vi "9234_Initialize.vi"(8 "error in (no error)":errorcluster, 9 "Slot Settings":T1, 11 "9234 in":refnum<class "9234.lvclass">) -> (0 "error out":errorcluster, 3 "9234 out":refnum<class "9234.lvclass">)   [LabVIEW 2017, in "Modules.lvlib" / "9234.lvclass"]
uses:
  9234.lvclass
  RSI Module/Slot Settings.ctl
  C:/Users/dbuck/Documents/GitHub/Scan-Engine-Custom-Device-Classes/Source/RSI Module/RSI Module.lvclass
  RSI Module/Channels.ctl
  RSI Module/Channel Type.ctl
  RSI Module/Module Models.ctl
  Data rate.ctl
  9234.lvclass/9234.ctl
  RSI Module/RSI Module.lvclass
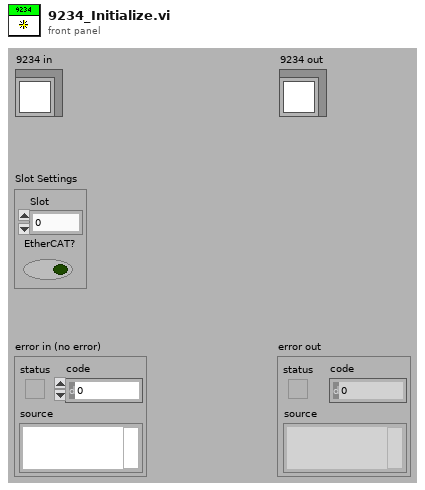
[diagram p1: front panel]
types:
  T1 = typedef "Modules.lvlib/RSI Module.lvclass/Slot Settings.ctl" = cluster{"Slot":u32, "EtherCAT?":bool}
  T2 = typedef "Modules.lvlib/RSI Module.lvclass/Module Models.ctl" = enum16{"Empty", "NI 9201", "NI 9203", "NI 9205", "NI 9206", "NI 9207", "NI 9208", "NI 9211", "NI 9212", "NI 9213", "NI 9214", "NI 9215", "NI 9217", "NI 9219", "NI 9220", "NI 9221", "NI 9222", "NI 9223", "NI 9225", "NI 9227", "NI 9229", "NI 9233", "NI 9234", "NI 9235", "NI 9236", "NI 9237", "NI 9239", "NI 9242", "NI 9244", "NI 9263", "NI 9264", "NI 9265", "NI 9269", "NI 9375", "NI 9401", "NI 9402", "NI 9403", "NI 9411", "NI 9421", "NI 9422", "NI 9423", "NI 9425", "NI 9426", "NI 9435", "NI 9437", "NI 9472", "NI 9474", "NI 9475", "NI 9476", "NI 9477", "NI 9478", "NI 9481", "NI 9482", "NI 9485"}
  T3 = typedef "Modules.lvlib/9234.lvclass/Data rate.ctl" = u32
  T4 = typedef "Modules.lvlib/RSI Module.lvclass/Channels.ctl" = cluster{"# Input Channels":i32, "# Output Channels":i32, "Channel Type":T5, "Units":string}
  T5 = typedef "Modules.lvlib/RSI Module.lvclass/Channel Type.ctl" = enum16{"Analog", "Digital"}
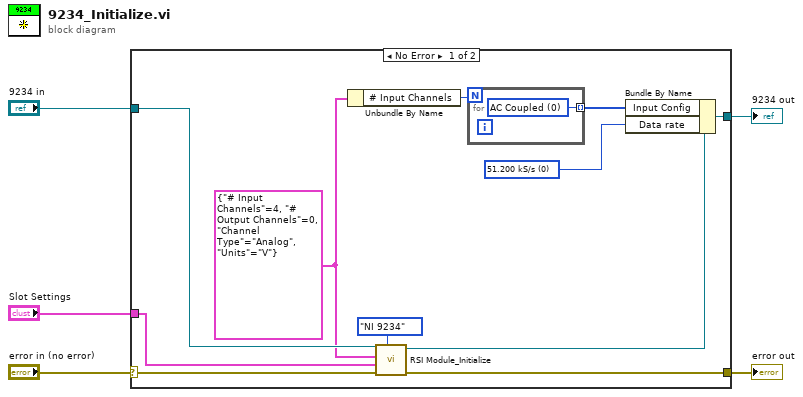
[diagram p0: block diagram]
diagram:
  n1 = case shown="No Error" "error in (no error)" {
    selector: "error in (no error)" -> [w14 w19]
    tunnel: [w13 w19] -> w4
    tunnel: [w11 w18] -> w2
    tunnel: "9234 in" -> [w16 w18]
    tunnel: "Slot Settings" -> [w15 _]
    frame No Error {
      w6 = T3 0 items=["51.200 kS/s", "25.600 kS/s", "17.067 kS/s", "12.800 kS/s", "10.240 kS/s", "8.533 kS/s", "7.314 kS/s", "6.400 kS/s", "5.689 kS/s", "5.120 kS/s", "4.654 kS/s", "4.267 kS/s", "3.938 kS/s", "3.657 kS/s", "3.413 kS/s", "3.200 kS/s", "3.012 kS/s", "2.845 kS/s", "2.695 kS/s", "2.560 kS/s", "2.438 kS/s", "2.328 kS/s", "2.226 kS/s", "2.133 kS/s", "2.048 kS/s", "1.969 kS/s", "1.896 kS/s", "1.829 kS/s", "1.765 kS/s", "1.707 kS/s", "1.652 kS/s"] ("Data rate")
      w9 = T4 {"# Input Channels"=4, "# Output Channels"=0, "Channel Type"=enum."Analog", "Units"="V"} ("Channels")
      n2 = Unbundle By Name(w9) -> ("# Input Channels"=w8:i32)
      n3 = call "RSI Module_Initialize.vi"("Module Model"=Module_Models."NI 9234", "error in (no error)"=w14, "Slot Settings"=w15, "Channels"=w9, "RSI Module in"=w16) -> ("error out"=w13:errorcluster, "RSI Module out"=w12:refnum<class "9234.lvclass">)  [unwired: 5 in]
      n4 = for {
        N: w8 -> [_]
        tunnel: [w17] -> w7 mode=indexing
        w17 = u32 0 items=["AC Coupled", "DC Coupled", "IEPE AC Coupled"] ("Input configuration")
      }
      n5 = Bundle By Name(cluster=w12, "Input Config"=w7, "Data rate"=w6) -> (w11:refnum<class "9234.lvclass">)
    }
    frame Error {
    }
  }
  "error out" <- w4
  "9234 out" <- w2
